vi "Solution part 2.vi"() -> ()   [LabVIEW 2020]
panel:
  out "result":i32
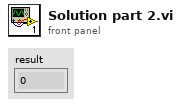
[diagram p1: front panel]
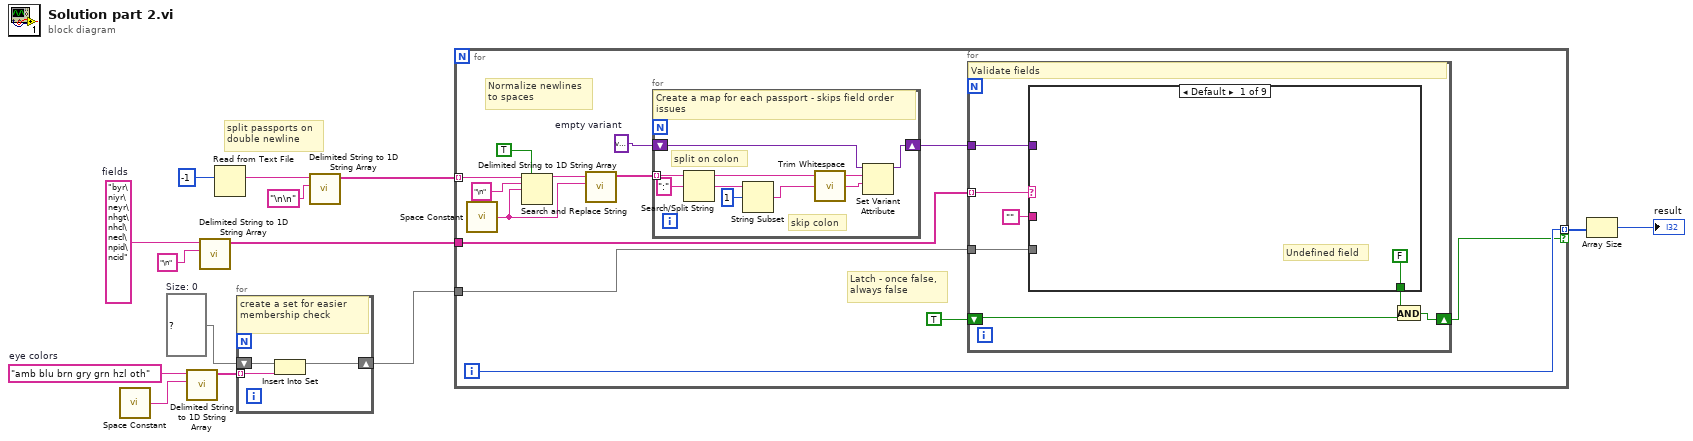
[diagram p0: block diagram]
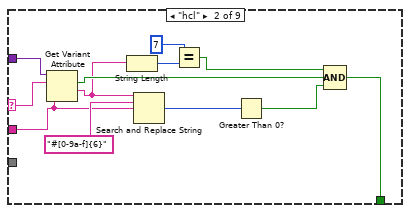
[diagram p2: hidden frame]
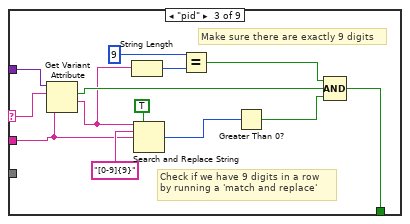
[diagram p3: hidden frame]
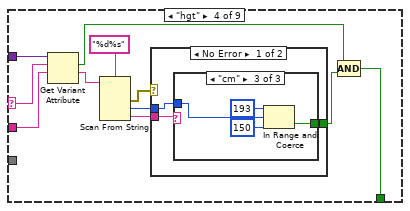
[diagram p4: hidden frame]
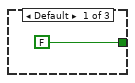
[diagram p5: hidden frame]
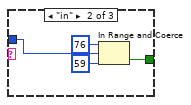
[diagram p6: hidden frame]
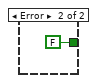
[diagram p7: hidden frame]
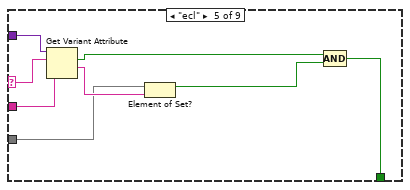
[diagram p8: hidden frame]
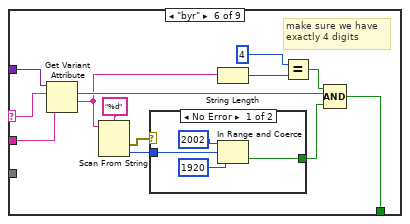
[diagram p9: hidden frame]
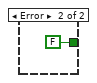
[diagram p10: hidden frame]
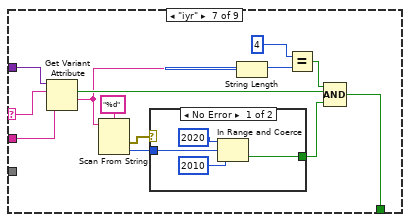
[diagram p11: hidden frame]
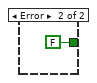
[diagram p12: hidden frame]
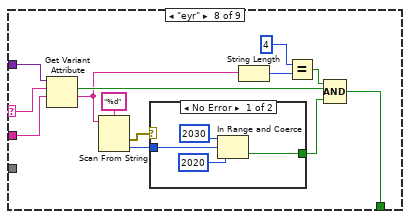
[diagram p13: hidden frame]
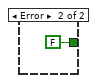
[diagram p14: hidden frame]
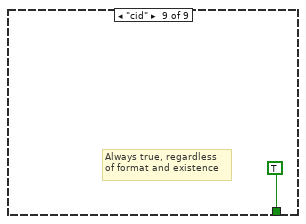
[diagram p15: hidden frame]
diagram:
  w2 = set{string} {}  # Size: 0
  w5 = "amb blu brn gry grn hzl oth"  # eye colors
  w8 = "byr\niyr\neyr\nhgt\nhcl\necl\npid\ncid"  # fields
  # "split passports on \ndouble newline"
  n1 = call <vilib>:"Space Constant.vi"() -> ("String"=w4:string)
  n2 = call <vilib>:"Delimited String to 1D String Array.vi"("delimiter"=w4, "delimited string"=w5) -> ("string array"=w3:string[])  [unwired: 9 in]
  n3 = call <vilib>:"Delimited String to 1D String Array.vi"("delimiter"="\n", "delimited string"=w8) -> ("string array"=w6:string[])  [unwired: 9 in]
  n4 = Read from Text File(count=-1) -> (text=w11:string)  [unwired: 3 in, 3 out]
  n5 = for {
    tunnel: w3 -> [w17] mode=indexing
    shift-right: [w15] -> w1
    shift-left: w2 -> [w16]
    # "create a set for easier membership check"
    n6 = Insert Into Set(10:w17, 11:w16) -> (3:w15:set{string})  [unwired: 1 out]
  }
  n7 = call <vilib>:"Delimited String to 1D String Array.vi"("delimiter"="\n\n", "delimited string"=w11) -> ("string array"=w10:string[])  [unwired: 9 in]
  n8 = for {
    tunnel: w10 -> [w29] mode=indexing
    tunnel: [w30] -> w14 mode=indexing if=w20
    tunnel: w6 -> [w23]
    tunnel: w1 -> [w18]
    i -> [w30]
    w24 = variant  # empty variant
    # "Latch - once false,\nalways false"
    # "Normalize newlines\nto spaces"
    n9 = call <vilib>:"Space Constant.vi"() -> ("String"=w26:string)
    n10 = Search and Replace String(replace all?=TRUE ("replace all? (F)"), input string=w29, search string="\n", replace string=w26) -> (result string=w27:string)  [unwired: 4 in, 3 out]
    n11 = call <vilib>:"Delimited String to 1D String Array.vi"("delimiter"=w26, "delimited string"=w27) -> ("string array"=w25:string[])  [unwired: 9 in]
    n12 = for {
      tunnel: w25 -> [w159] mode=indexing
      shift-right: [w154] -> w22
      shift-left: w24 -> [w155]
      # "split on colon"
      # "skip colon"
      # "Create a map for each passport - skips field order issues"
      n13 = Search/Split String(string=w159, search string/char (-)=":") -> (substring before match=w156:string, match + rest of string=w153:string)  [unwired: 1 in, 1 out]
      n14 = String Subset(string=w153, offset (0)=1) -> (substring=w152:string)  [unwired: 1 in]
      n15 = call <vilib>:"Trim Whitespace.vi"("string"=w152) -> ("trimmed string"=w157:string)  [unwired: 1 in]
      n16 = Set Variant Attribute(Variant=w155, name=w156, value=w157) -> (Variant out=w154:variant)  [unwired: 1 in, 2 out]
    }
    n17 = for {
      tunnel: w23 -> [w33] mode=indexing
      tunnel: w22 -> [w34]
      shift-right: [w36] -> w20
      shift-left: TRUE -> [w37]
      tunnel: w18 -> [w31]
      # "Validate fields"
      n18 = case shown="Default" w33 {
        selector: w33 -> [_ w49 w62 w73 w94 w107 w125 w143 _]
        tunnel: [FALSE w48 w61 w71 w92 w104 w122 w140 TRUE] -> w35
        tunnel: w34 -> [_ w50 w63 w74 w95 w108 w126 w144 _]
        tunnel: "" -> [_ w45 w58 w72 w93 w106 w124 w142 _]
        tunnel: w31 -> [_ _ _ _ w89 _ _ _ _]
        frame Default {
          # "Undefined field"
        }
        frame "hcl" {
          n19 = Get Variant Attribute(Variant=w50, name=w49, default value (empty Variant)=w45) -> (found=w47:bool, value=w41:string)  [unwired: 1 in, 2 out]
          n20 = String Length(string=w41) -> (length=w42:i32)
          n21 = Search and Replace String(input string=w41, search string="#[0-9a-f]{6}" ("regular expression"), replace string=w45) -> (number of replacements=w44:i32)  [unwired: 5 in, 3 out]
          n22 = Equal?(x=7, y=w42) -> (x = y?=w39:bool)
          n23 = Greater Than 0?(x=w44) -> (x > 0?=w43:bool)
          n24 = Compound Arithmetic op=AND(w39, w47, w43) -> (w48:bool)
        }
        frame "pid" {
          # "Make sure there are exactly 9 digits"
          # "Check if we have 9 digits in a row\nby running a 'match and replace'"
          n25 = Get Variant Attribute(Variant=w63, name=w62, default value (empty Variant)=w58) -> (found=w60:bool, value=w53:string)  [unwired: 1 in, 2 out]
          n26 = String Length(string=w53) -> (length=w55:i32)
          n27 = Search and Replace String(replace all?=TRUE ("replace all? (F)"), input string=w53, search string="[0-9]{9}" ("regular expression"), replace string=w58) -> (number of replacements=w57:i32)  [unwired: 4 in, 3 out]
          n28 = Equal?(x=9, y=w55) -> (x = y?=w52:bool)
          n29 = Greater Than 0?(x=w57) -> (x > 0?=w56:bool)
          n30 = Compound Arithmetic op=AND(w52, w60, w56) -> (w61:bool)
        }
        frame "hgt" {
          n31 = Get Variant Attribute(Variant=w74, name=w73, default value (empty Variant)=w72) -> (found=w70:bool, value=w69:string)  [unwired: 1 in, 2 out]
          n32 = Scan From String(format string="%d%s", input string=w69) -> (error out=w64:errorcluster, output 1=w65:i32, output 2=w67:string)  [unwired: 4 in, 2 out]
          n33 = case shown="No Error" w64 {
            tunnel: w67 -> [w77 _]
            tunnel: [w76 FALSE] -> w66
            tunnel: w65 -> [w75 _]
            frame No Error {
              n34 = case shown="\"cm\"" w77 {
                tunnel: [FALSE w82 w86] -> w76
                tunnel: w75 -> [_ w81 w85]
                frame Default {
                }
                frame "in" {
                  n35 = In Range and Coerce(upper limit=76, x=w81, lower limit=59) -> (In Range?=w82:bool)  [unwired: 1 out]
                }
                frame "cm" {
                  n36 = In Range and Coerce(upper limit=193, x=w85, lower limit=150) -> (In Range?=w86:bool)  [unwired: 1 out]
                }
              }
            }
            frame Error {
            }
          }
          n37 = Compound Arithmetic op=AND(w70, w66) -> (w71:bool)
        }
        frame "ecl" {
          n38 = Get Variant Attribute(Variant=w95, name=w94, default value (empty Variant)=w93) -> (found=w91:bool, value=w90:string)  [unwired: 1 in, 2 out]
          n39 = Element of Set?(10:w90, 11:w89) -> (3:w88:bool)
          n40 = Compound Arithmetic op=AND(w91, w88) -> (w92:bool)
        }
        frame "byr" {
          # "make sure we have \nexactly 4 digits"
          n41 = Get Variant Attribute(Variant=w108, name=w107, default value (empty Variant)=w106) -> (found=w105:bool, value=w100:string)  [unwired: 1 in, 2 out]
          n42 = Scan From String(format string="%d", input string=w100) -> (error out=w98:errorcluster, output 1=w97:i32)  [unwired: 3 in, 2 out]
          n43 = case shown="No Error" w98 {
            tunnel: w97 -> [w110 _]
            tunnel: [w109 FALSE] -> w96
            frame No Error {
              n44 = In Range and Coerce(upper limit=2002, x=w110, lower limit=1920) -> (In Range?=w109:bool)  [unwired: 1 out]
            }
            frame Error {
            }
          }
          n45 = String Length(string=w100) -> (length=w103:i32)
          n46 = Equal?(x=4, y=w103) -> (x = y?=w101:bool)
          n47 = Compound Arithmetic op=AND(w101, w105, w96) -> (w104:bool)
        }
        frame "iyr" {
          n48 = Get Variant Attribute(Variant=w126, name=w125, default value (empty Variant)=w124) -> (found=w123:bool, value=w118:string)  [unwired: 1 in, 2 out]
          n49 = Scan From String(format string="%d", input string=w118) -> (error out=w116:errorcluster, output 1=w115:i32)  [unwired: 3 in, 2 out]
          n50 = case shown="No Error" w116 {
            tunnel: w115 -> [w128 _]
            tunnel: [w127 FALSE] -> w114
            frame No Error {
              n51 = In Range and Coerce(upper limit=2020, x=w128, lower limit=2010) -> (In Range?=w127:bool)  [unwired: 1 out]
            }
            frame Error {
            }
          }
          n52 = String Length(string=w118) -> (length=w121:i32)
          n53 = Equal?(x=4, y=w121) -> (x = y?=w119:bool)
          n54 = Compound Arithmetic op=AND(w119, w123, w114) -> (w122:bool)
        }
        frame "eyr" {
          n55 = Get Variant Attribute(Variant=w144, name=w143, default value (empty Variant)=w142) -> (found=w141:bool, value=w136:string)  [unwired: 1 in, 2 out]
          n56 = Scan From String(format string="%d", input string=w136) -> (error out=w134:errorcluster, output 1=w133:i32)  [unwired: 3 in, 2 out]
          n57 = case shown="No Error" w134 {
            tunnel: w133 -> [w146 _]
            tunnel: [w145 FALSE] -> w132
            frame No Error {
              n58 = In Range and Coerce(upper limit=2030, x=w146, lower limit=2020) -> (In Range?=w145:bool)  [unwired: 1 out]
            }
            frame Error {
            }
          }
          n59 = String Length(string=w136) -> (length=w139:i32)
          n60 = Equal?(x=4, y=w139) -> (x = y?=w137:bool)
          n61 = Compound Arithmetic op=AND(w137, w141, w132) -> (w140:bool)
        }
        frame "cid" {
          # "Always true, regardless\nof format and existence"
        }
      }
      n62 = And(x=w35, y=w37) -> (x .and. y?=w36:bool)
    }
  }
  n63 = Array Size(array=w14) -> (size(s)=→"result":i32)
